vi "MT_GET.vi"(8 "Use checksum":bool, 11 "read buffer":string) -> (0 "MT check sum":u8, 1 "sample counter":i16, 2 "MT_DATA":sgl[](array[numeric]), 4 "MT_BITS":u8[](array[numeric]))   [LabVIEW 2014]
uses:
  <vilib>/imath/engines/lvmath2/RunTimeEngine/BuiltInFunctions/length/NIMS_length(GV).vi
  <instcachedir>/0/NIMS_length(GV)_08A3D13377FD4E4B96F5795FBF3698FA.lvgen/NIMS_length(GV)_08A3D13377FD4E4B96F5795FBF3698FA_003.vi
  <vilib>/imath/engines/lvmath2/RunTimeEngine/RangeToken/NIMS_Range_R2 - Integer.vi
  <instcachedir>/0/NIMS_Range_R2 - Integer_2D1304BAF97744E0A293025746CBADFC.lvgen/NIMS_Range_R2 - Integer_2D1304BAF97744E0A293025746CBADFC_000.vi
  <vilib>/imath/engines/lvmath2/RunTimeEngine/CommandStatement/MC_CommandStatement_break.vi
  <vilib>/imath/engines/lvmath2/RunTimeEngine/IndexRead/NIMS V(S).vi
  <instcachedir>/0/NIMS V(S)_0488751826AF41519A22953C041130DC.lvgen/NIMS V(S)_0488751826AF41519A22953C041130DC_003.vi
  <vilib>/imathl/engines/lvmath/Functions/Error Handling/Create Error.vi
  <vilib>/imath/engines/lvmath2/RunTimeEngine/BuiltInFunctions/mod/NIMS_mod_no_size_check.vi
  <instcachedir>/0/NIMS_mod_no_size_check_5393E3382FD241D281EEB71DA286C65B.lvgen/NIMS_mod_no_size_check_5393E3382FD241D281EEB71DA286C65B_008.vi
  <vilib>/imath/engines/lvmath2/RunTimeEngine/BuiltInFunctions/uint8/NIMS_uint8(int).vi
  <instcachedir>/0/NIMS_uint8(int)_9D6EF81F86254677BB00410F9E5C6A1D.lvgen/NIMS_uint8(int)_9D6EF81F86254677BB00410F9E5C6A1D_000.vi
  <vilib>/imath/engines/lvmath2/RunTimeEngine/NodeEndStatement/NIMS_NodeEndStatement_Output.vi
  <instcachedir>/0/NIMS_NodeEndStatement_Output_53EC0D466D134D7ABD903AC30B43404B.lvgen/NIMS_NodeEndStatement_Output_53EC0D466D134D7ABD903AC30B43404B_013.vi
  <instcachedir>/0/NIMS_NodeEndStatement_Output_53EC0D466D134D7ABD903AC30B43404B.lvgen/NIMS_NodeEndStatement_Output_53EC0D466D134D7ABD903AC30B43404B_012.vi
  <vilib>/imath/engines/lvmath2/RunTimeEngine/ErrorHandling/NIMS_Finalize Error.vi
panel:
  out "New checksum":u8
  out "New checksum OK?":bool
  out "size(s)":i32
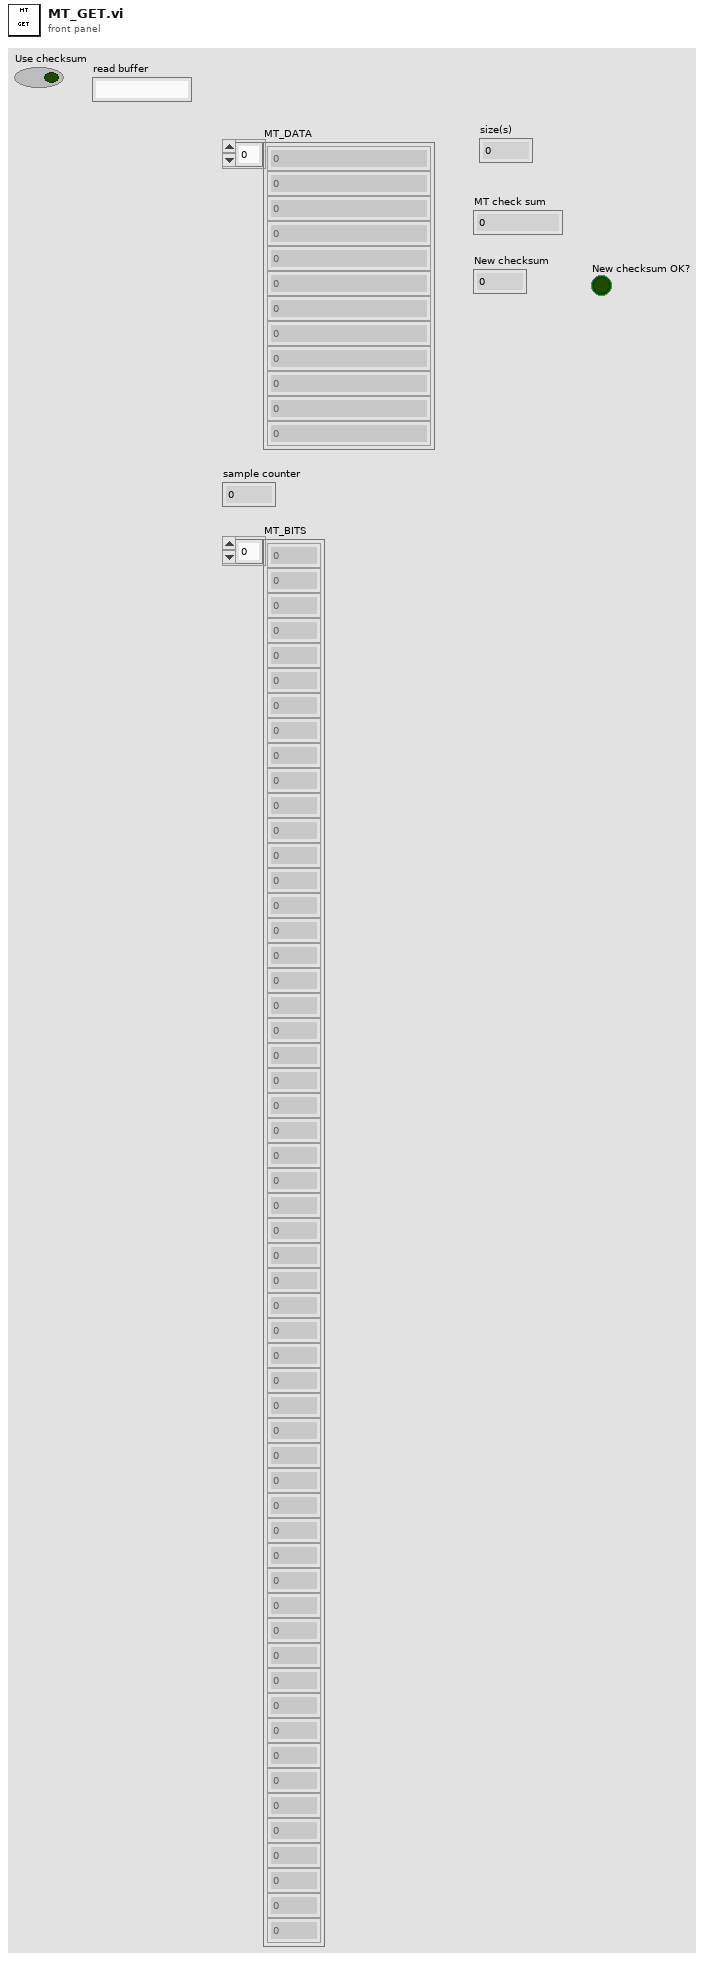
[diagram p1: front panel]
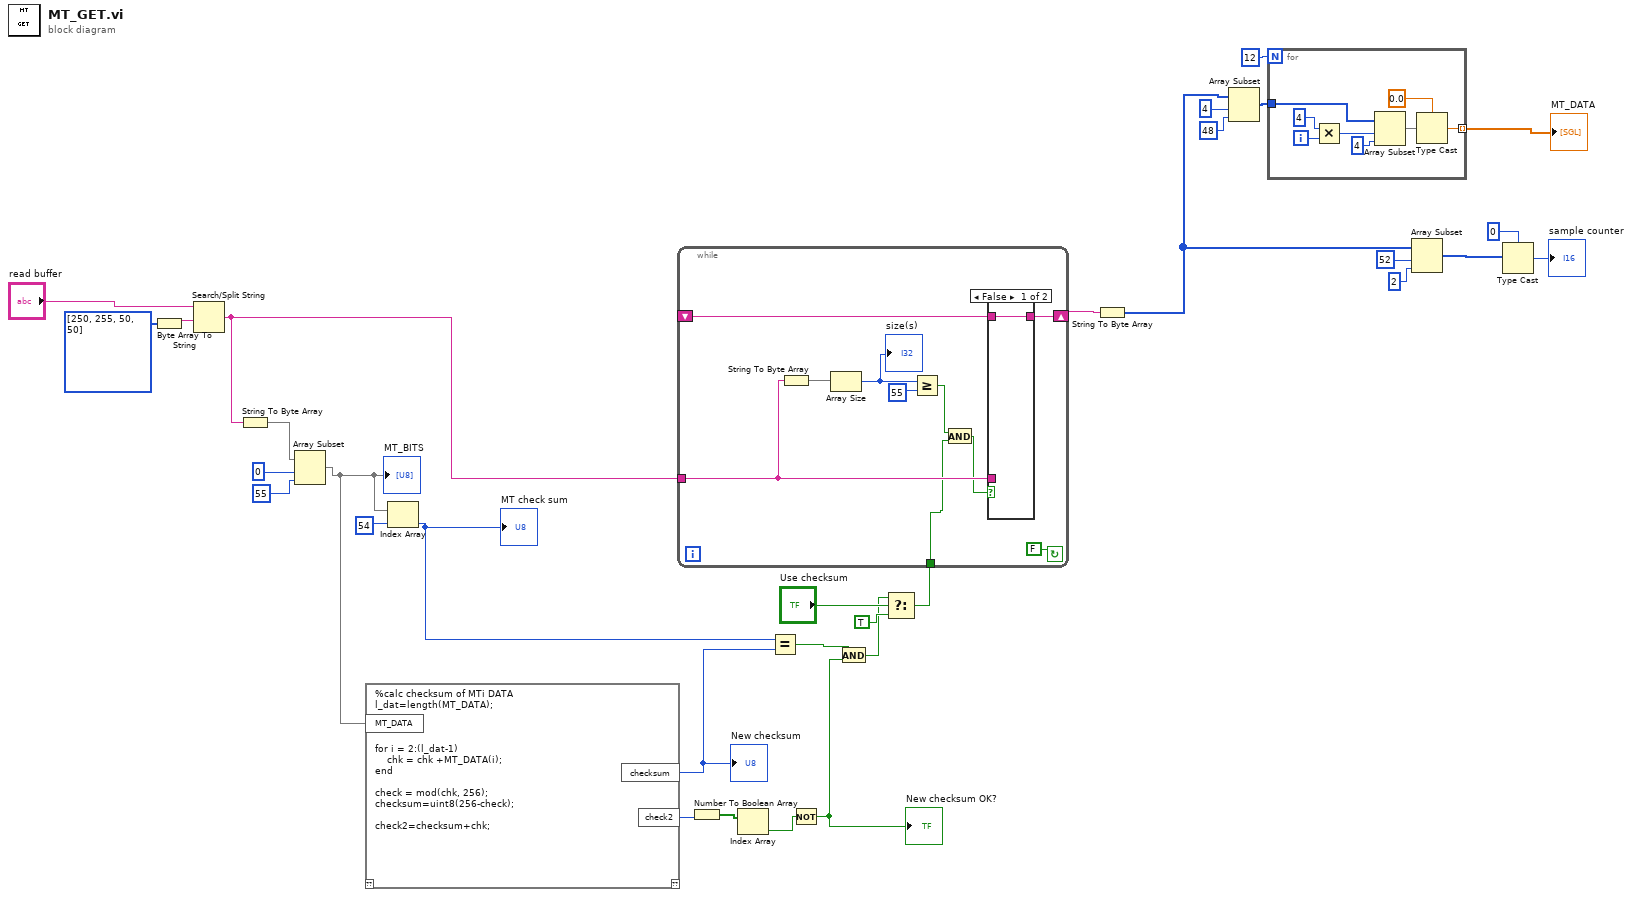
[diagram p0: block diagram]
diagram:
  n1 = Byte Array To String(unsigned byte array=u8[] [250, 255, 50, 50]) -> (string=w32:string)
  n2 = Search/Split String(string="read buffer", search string/char (-)=w32) -> (match + rest of string=w14:string)  [unwired: 1 in, 2 out]
  n3 = String To Byte Array(string=w14) -> (unsigned byte array=w13:u8[])
  n4 = Array Subset(array=w13, index=0, length=55) -> (w12:u8[])
  "MT_BITS" <- w12
  n5 = mathscript code="%calc checksum of MTi DATA\nl_dat=length(MT_DATA);\n\nchk = 0;\n\nfor i = 2:(l_dat-1)\n    chk = chk +MT_DATA(i);\nend\n\ncheck = mod(chk, 256);\nchecksum=uint8(256-check);\n\ncheck2=checksum+chk;"("MT_DATA"=w12) -> ("checksum"=w10:u8, "check2"=w9:i32)  [unwired: 1 in, 1 out]
  "New checksum" <- w10
  n6 = Index Array(array=w12, index=54) -> (element=w11:u8)
  "MT check sum" <- w11
  n7 = Number To Boolean Array(number=w9) -> (Boolean array=w8:bool[])
  n8 = Index Array(array=w8) -> (element=w7:bool)  [unwired: 1 in]
  n9 = Equal?(x=w11, y=w10) -> (x = y?=w6:bool)
  n10 = Not(x=w7) -> (.not. x?=w5:bool)
  "New checksum OK?" <- w5
  n11 = And(x=w6, y=w5) -> (x .and. y?=w2:bool)
  n12 = Select(t=w2, s="Use checksum", f=TRUE) -> (s? t:f=w1:bool)
  n13 = while {
    tunnel: w14 -> [w38]
    shift-right: [w37] -> w17
    shift-left: _ -> [w36]
    tunnel: w1 -> [w33]
    stop <- FALSE continue-if-true
    n14 = String To Byte Array(string=w38) -> (unsigned byte array=w41:u8[])
    n15 = Array Size(array=w41) -> (size(s)=w40:i32)
    "size(s)" <- w40
    n16 = Greater Or Equal?(x=w40, y=55) -> (x >= y?=w35:bool)
    n17 = And(x=w35, y=w33) -> (x .and. y?=w34:bool)
    n18 = case shown="False" w34 {
      tunnel: w38 -> [_ w44]
      tunnel: [w43 w44] -> w37
      tunnel: w36 -> [w43 _]
      frame False {
      }
      frame True {
      }
    }
  }
  n19 = String To Byte Array(string=w17) -> (unsigned byte array=w18:u8[])
  n20 = Array Subset(array=w18, index=4, length=48) -> (w23:u8[])
  n21 = for {
    N: 12 -> [_]
    tunnel: w23 -> [w47]
    tunnel: [w45] -> w30 mode=indexing
    i -> [w50]
    n22 = Multiply(x=4 ("index"), y=w50) -> (x*y=w48:i32)
    n23 = Array Subset(array=w47, index=w48, length=4) -> (w46:u8[])
    n24 = Type Cast(type=sgl 0.0, x=w46) -> (*(type *) &x=w45:sgl)
  }
  "MT_DATA" <- w30
  n25 = Array Subset(array=w18, index=52, length=2) -> (w28:u8[])
  n26 = Type Cast(type=i16 0, x=w28) -> (*(type *) &x=→"sample counter":i16)
